vi "Calc_Exec_Time_vs_CuLab.vi"(11 "Exec Times":cluster{"Array":i32[], "all rows":dbl[]}[](array[cluster])) -> (0 "Mean Gain":dbl[](array[numeric]), 3 "CuLab Gain":cluster{"Array":i32[], "all rows":dbl[]}[](array[cluster]))   [LabVIEW 2020]
uses:
  <vilib>/Analysis/baseanly.llb/Mean (DBL).vi
  <vilib>/Analysis/NI_AALBase.lvlib
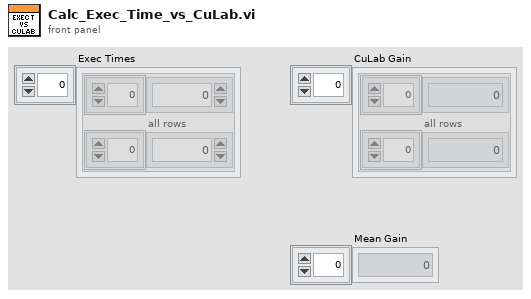
[diagram p1: front panel]
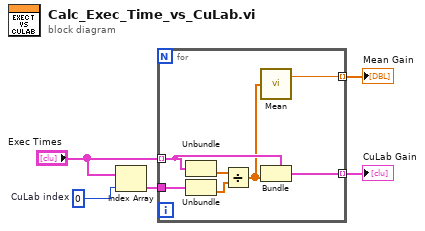
[diagram p0: block diagram]
diagram:
  w2 = 0  # CuLab index
  n1 = Index Array(array="Exec Times", index=w2) -> (element=w1:cluster{"Array":i32[], "all rows":dbl[]})
  n2 = for {
    tunnel: "Exec Times" -> [w12] mode=indexing
    tunnel: w1 -> [w10]
    tunnel: [w11] -> w3 mode=indexing
    tunnel: [w6] -> w4 mode=indexing
    n3 = Unbundle(w12) -> ("all rows"=w9:dbl[])  [unwired: 1 out]
    n4 = Unbundle(w10) -> ("all rows"=w8:dbl[])  [unwired: 1 out]
    n5 = Divide(x=w9, y=w8) -> (x/y=w7:dbl[])
    n6 = call-poly <vilib>:"Mean.vi"("X"=w7) -> ("mean"=w6:dbl)  [unwired: 1 out]
    n7 = Bundle(cluster=w12, "all rows"=w7) -> (w11:cluster{"Array":i32[], "all rows":dbl[]})  [unwired: 1 in]
  }
  "Mean Gain" <- w4
  "CuLab Gain" <- w3
